vi "Init.vi"(8 "error in (no error)":errorcluster, 11 "Execution API In":refnum<class "Execution API.lvclass">) -> (0 "error out":errorcluster, 3 "Execution API Out":refnum<class "Execution API.lvclass">)   [LabVIEW 2020]
doc: "Initializes the process and creates necessary references. Anything initialized here is released in the Clear.vi method."
uses:
  Execution API.lvclass
  Core/Result/Result.ctl
  Core/Result/Status.ctl
  Core/Result/Type.ctl
  Execution API.lvclass/Execution API.ctl
  Core/Result/Result.lvlib
  C:/git/astemes-lunit/source/User Interface/Execution API/Execution API.lvclass
  C:/git/astemes-lunit/source/Framework/Result Observer/Result Observer.lvclass
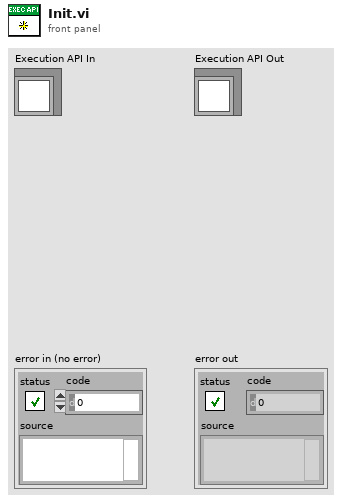
[diagram p1: front panel]
types:
  T1 = typedef "Result.lvlib/Result.ctl" = cluster{"Name":string, "Message":string, "Description":string, "Status":T2, "Result Type":T3, "Execution Time":dbl}
  T2 = typedef "Result.lvlib/Status.ctl" = enum16{"", "Passed", "Failed", "Error", "Skipped", "Setup Error", "Broken", "Teardown Error"}
  T3 = typedef "Result.lvlib/Type.ctl" = enum16{"Method", "Case", "Suite", "Pass", "Fail", "Skip", "Pass if", "Fail if", "Pass if Error", "Fail if Error", "Pass if Equal", "Fail if Equal"}
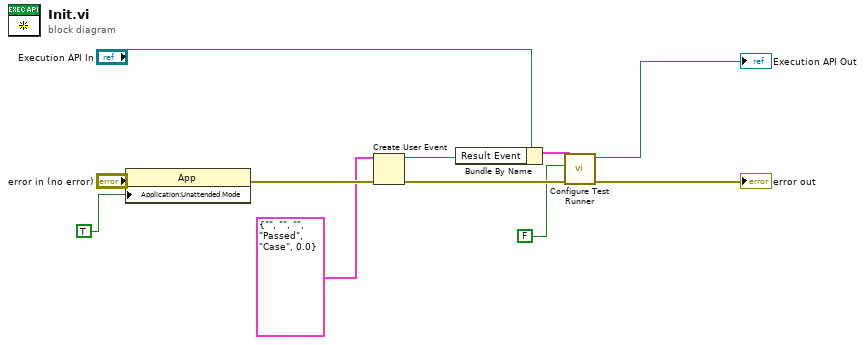
[diagram p0: block diagram]
diagram:
  n1 = property class="App"(error in="error in (no error)", "Application:Unattended Mode"=TRUE) -> (error out=w9:errorcluster)  [unwired: 1 in, 1 out]
  n2 = Create User Event(user event datatype=T1 {"Name"="", "Message"="", "Description"="", "Status"=enum."Passed", "Result Type"=enum."Case", "Execution Time"=0.0} ("Result"), error in=w9) -> (user event=w6:refnum<user-event>, error out=w7:errorcluster)
  n3 = Bundle By Name(cluster="Execution API In", "Result Event"=w6) -> (w4:cluster{})
  n4 = call "Configure Test Runner.vi"("error in (no error)"=w7, "Run Tests In Parallel?"=FALSE, "Execution API In"=w4) -> ("error out"=→"error out":errorcluster, "Execution API Out"=→"Execution API Out":refnum<class "Execution API.lvclass">)  [unwired: 7 in]
